vi "test Fit Scale Range to Content 1.vi"(11 "Test Case In":refnum<class "test Fit Scale Range to Content.lvclass">) -> (0 "error out":errorcluster, 3 "Test Case Out":refnum<class "test Fit Scale Range to Content.lvclass">)   [LabVIEW 2023, in "test Fit Scale Range to Content.lvclass"]
uses:
  test Fit Scale Range to Content.lvclass
  C:/Program Files/National Instruments/LabVIEW 2023/vi.lib/Astemes/LUnit/Test Case.lvclass
  source/Base Graph/Base Graph.lvclass/Base Graph.ctl
  <vilib>/Astemes/LUnit/Test Case.lvclass/Test Case.ctl
  <vilib>/Astemes/LUnit/Append Fail Result.vi
  <vilib>/Astemes/LUnit/Append Pass Result.vi
  <vilib>/Astemes/LUnit/Run In UI.vi
  <vilib>/Utility/error.llb/Clear Errors.vi
  <vilib>/Analysis/Matrix/Numeric/Conversions/Array To Matrix - RA2.vi
  test Fit Scale Range to Content.lvclass/test Fit Scale Range to Content.ctl
  source/Base Graph/Base Graph.lvclass
  <vilib>/Analysis/Matrix/NI_Matrix.lvlib
  <vilib>/Astemes/LUnit/Test Case.lvclass
panel:
  out "Intensity Graph":dbl[][](graph)
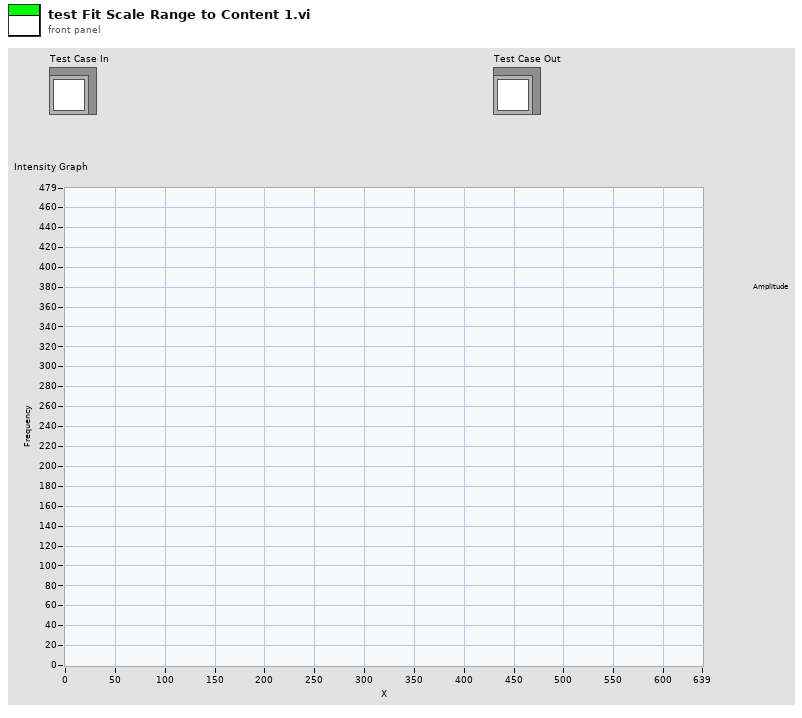
[diagram p1: front panel]
types:
  T1 = typedef "NI_Matrix.lvlib/RealMatrix.ctl" = dbl[][]
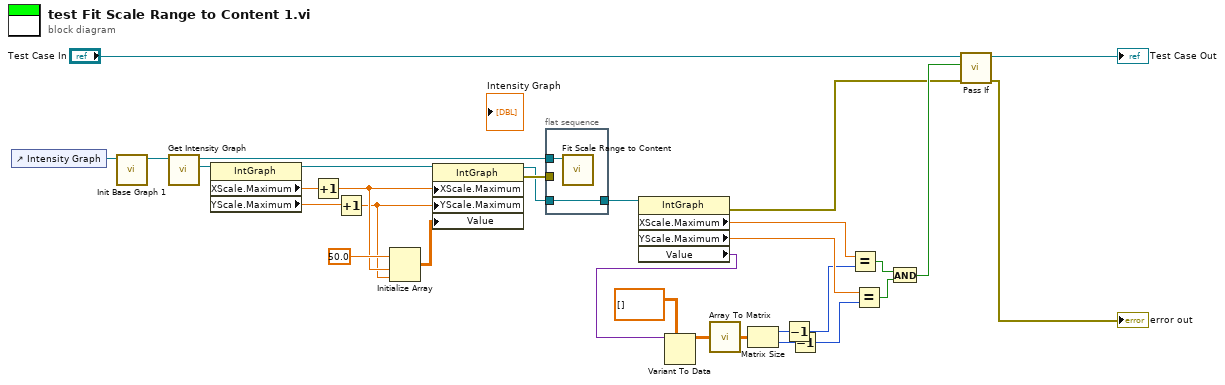
[diagram p0: block diagram]
diagram:
  n1 = control-ref of="Intensity Graph"() -> (w28:refnum<vi>)
  n2 = call "Init Base Graph 1.vi"("IntensityGraph in"=w28) -> ("Base Graph out"=w27:refnum<class "Base Graph.lvclass">)  [unwired: 10 in]
  n3 = call "Get Intensity Graph.vi"("Base Graph in"=w27) -> ("Intensity Graph"=w25:refnum<vi>, "Base Graph out"=w26:refnum<class "Base Graph.lvclass">)  [unwired: 9 in]
  n4 = property class="IntGraph"(reference=w25) -> (reference out=w24:refnum<vi>, "XScale.Maximum"=w6:dbl, "YScale.Maximum"=w5:dbl)  [unwired: 1 in, 1 out]
  n5 = Increment(x=w6) -> (x+1=w4:dbl)
  n6 = Increment(x=w5) -> (x+1=w3:dbl)
  n7 = Initialize Array(50.0 ("element"), w4, w3) -> (w8:dbl[][])
  n8 = property class="IntGraph"(reference=w24, "XScale.Maximum"=w4, "YScale.Maximum"=w3, "Value"=w8) -> (reference out=w21:refnum<vi>, error out=w23:errorcluster)  [unwired: 1 in]
  n9 = flat-sequence {
    tunnel: w26 -> [w33]
    tunnel: w23 -> [_]
    tunnel: [w32] -> w22
    tunnel: w21 -> [w32]
    frame #0 {
      n10 = call "Fit Scale Range to Content.vi"("Base Graph in"=w33) -> ()  [unwired: 10 in, 1 out]
    }
  }
  n11 = property class="IntGraph"(reference=w22) -> (error out=w10:errorcluster, "XScale.Maximum"=w17:dbl, "YScale.Maximum"=w15:dbl, "Value"=w9:variant)  [unwired: 1 in, 1 out]
  n12 = Variant To Data(type=dbl[][] [], Variant=w9) -> (data=w19:dbl[][])  [unwired: 1 in, 1 out]
  n13 = call-poly <vilib>:"Array To Matrix.vi"("Real 2D Array"=w19) -> ("Real Matrix"=w18:T1)
  n14 = Matrix Size(0:w18) -> (1:w16:i32, 2:w14:i32)
  n15 = Decrement(x=w16) -> (x-1=w2:i32)
  n16 = Decrement(x=w14) -> (x-1=w1:i32)
  n17 = Equal?(x=w17, y=w2) -> (x = y?=w13:bool)
  n18 = Equal?(x=w15, y=w1) -> (x = y?=w12:bool)
  n19 = And(x=w13, y=w12) -> (x .and. y?=w11:bool)
  n20 = call <vilib>:"Pass If.vi"("error in (no error)"=w10, "Pass?"=w11, "LUnit Test Case In"="Test Case In") -> ("error out"=→"error out":errorcluster, "LUnit Test Case Out"=→"Test Case Out":refnum<class "test Fit Scale Range to Content.lvclass">)  [unwired: 7 in]
